vi "FirmwareVer 2 Case (uSMC).vi"(1 "SMindex":i32) -> (0 "Case":i32)   [LabVIEW 2010, in "SignalWriterMH110203USBStepperMotor.lvclass"]
uses:
  SignalWriterMH110203USBStepperMotor.lvclass
  class_data.vi
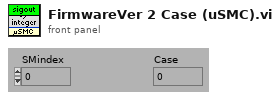
[diagram p1: front panel]
types:
  T1 = typedef "SignalWriterMH110203USBStepperMotor.lvclass/GoTo Control (uSMC).ctl" = cluster{"Step motor ID":string, "SMname":string, "Backlash":u16, "wait for input sygnal to start":bool, "use slow start/stop":bool, "units name":string, "Maximum speed":dbl, "speed":dbl, "step":u8, "point 1 ticks":i32, "point 2 ticks":i32, "point 1 units":dbl, "point 2 units":dbl, "Limit Switch standoff":dbl, "Zero Value":dbl, "Destination Position":dbl, "force backlash":bool, "power off when stop":bool, "POff delay":dbl, "positioner name":string, "R, Ohm":dbl, "I, mA":dbl, "Positioner's Type":u16, "Reset Direction":bool, "Manufacturer":string, "Model":string, "Scheme":string, "FirmwareVer":string}
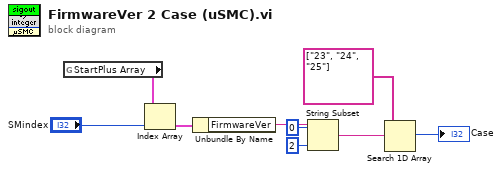
[diagram p0: block diagram]
diagram:
  n1 = global read "class_data.vi" "StartPlus Array"() -> (w1:T1[])
  n2 = Index Array(array=w1, index="SMindex") -> (element=w9:T1)
  n3 = Unbundle By Name(w9) -> ("FirmwareVer"=w7:string)
  n4 = String Subset(string=w7, offset (0)=0, length (rest)=2 ("length (rest)")) -> (substring=w4:string)
  n5 = Search 1D Array(1D array=string[] ["23", "24", "25"], element=w4) -> (index of element=→"Case":i32)  [unwired: 1 in]
